vi "BCD2String.vi"(11 "BCD Int":i64) -> (3 "String":string)   [LabVIEW 2020]
panel:
  out "hex integer string":string
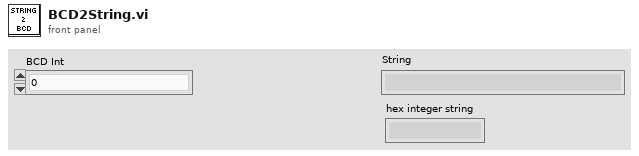
[diagram p1: front panel]
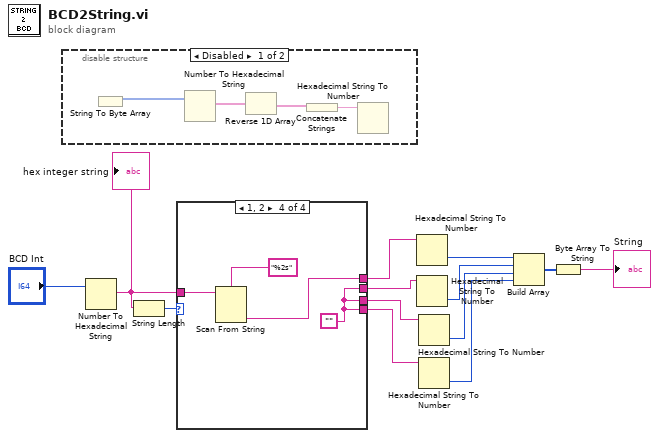
[diagram p0: block diagram]
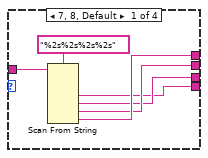
[diagram p2: hidden frame]
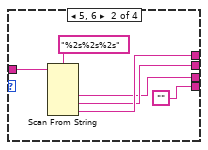
[diagram p3: hidden frame]
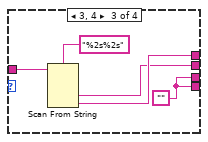
[diagram p4: hidden frame]
diagram:
  n1 = disable-structure shown="Disabled" {
    frame Disabled {
      n2 = String To Byte Array() -> (unsigned byte array=w17:u8[])  [unwired: 1 in]
      n3 = Number To Hexadecimal String(2:w17) -> (0:w15:string[])  [unwired: 1 in]
      n4 = Reverse 1D Array(array=w15) -> (reversed array=w14:string[])
      n5 = Concatenate Strings(w14) -> (w16:string)
      n6 = Hexadecimal String To Number(string=w16) -> ()  [unwired: 2 in, 2 out]
    }
    frame Enabled {
    }
  }
  n7 = Number To Hexadecimal String(2:"BCD Int") -> (0:w11:string)  [unwired: 1 in]
  "hex integer string" <- w11
  n8 = String Length(string=w11) -> (length=w12:i32)
  n9 = case shown="1, 2" w12 {
    tunnel: w11 -> [w23 w29 w34 w38]
    tunnel: [w21 w27 w32 w36] -> w7
    tunnel: [w20 w26 w31 w35] -> w8
    tunnel: [w19 w25 w30 w35] -> w9
    tunnel: [w18 "" w30 w35] -> w10
    frame 7, 8, Default {
      n10 = Scan From String(format string="%2s%2s%2s%2s", input string=w23) -> (output 1=w18:string, output 2=w19:string, output 3=w20:string, output 4=w21:string)  [unwired: 6 in, 3 out]
    }
    frame 5, 6 {
      n11 = Scan From String(format string="%2s%2s%2s", input string=w29) -> (output 1=w25:string, output 2=w26:string, output 3=w27:string)  [unwired: 5 in, 3 out]
    }
    frame 3, 4 {
      w30 = ""
      n12 = Scan From String(format string="%2s%2s", input string=w34) -> (output 1=w31:string, output 2=w32:string)  [unwired: 4 in, 3 out]
    }
    frame 1, 2 {
      w35 = ""
      n13 = Scan From String(format string="%2s", input string=w38) -> (output 1=w36:string)  [unwired: 3 in, 3 out]
    }
  }
  n14 = Hexadecimal String To Number(string=w7) -> (number=w6:u32)  [unwired: 2 in, 1 out]
  n15 = Hexadecimal String To Number(string=w8) -> (number=w5:u32)  [unwired: 2 in, 1 out]
  n16 = Hexadecimal String To Number(string=w9) -> (number=w4:u32)  [unwired: 2 in, 1 out]
  n17 = Hexadecimal String To Number(string=w10) -> (number=w3:u32)  [unwired: 2 in, 1 out]
  n18 = Build Array(w6, w5, w4, w3) -> (w2:u32[])
  n19 = Byte Array To String(unsigned byte array=w2) -> (string=→"String":string)
